vi "Refactor Class Dynamic Dispatch Membersvi.vi"(8 "error in (no error)":errorcluster, 10 "rename data in":T1, 11 "project classes in":refnum<vi>[](array[refnum])) -> (0 "error out":errorcluster, 1 "refactor results":T3[](array[typedef]), 2 "rename metadata out":T1, 3 "project classes out":refnum<vi>[](array[refnum]))   [LabVIEW 2020, in "MeasurementService Editor.lvlib"]
uses:
  MeasurementService Editor.lvlib
  Rename Refactor Data.ctl
  Rename Refactor Mapping Info.ctl
  Refactor Dynamic Dispatch Member Result.ctl
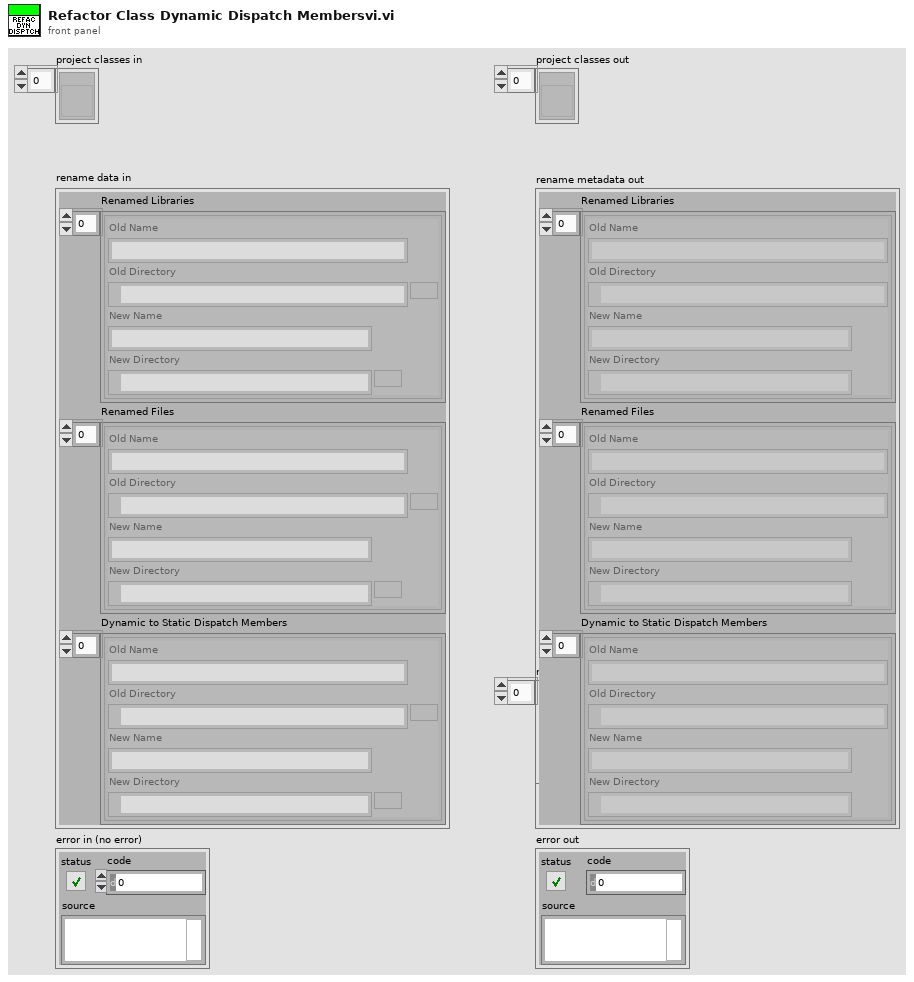
[diagram p1: front panel]
types:
  T1 = typedef "MeasurementService Editor.lvlib/Rename Refactor Data.ctl" = cluster{"Renamed Libraries":T2[], "Renamed Files":T2[], "Dynamic to Static Dispatch Members":T2[]}
  T2 = typedef "MeasurementService Editor.lvlib/Rename Refactor Mapping Info.ctl" = cluster{"Old Name":string, "Old Directory":path, "New Name":string, "New Directory":path}
  T3 = typedef "MeasurementService Editor.lvlib/Refactor Dynamic Dispatch Member Result.ctl" = cluster{"Old Path":path, "New Path":path}
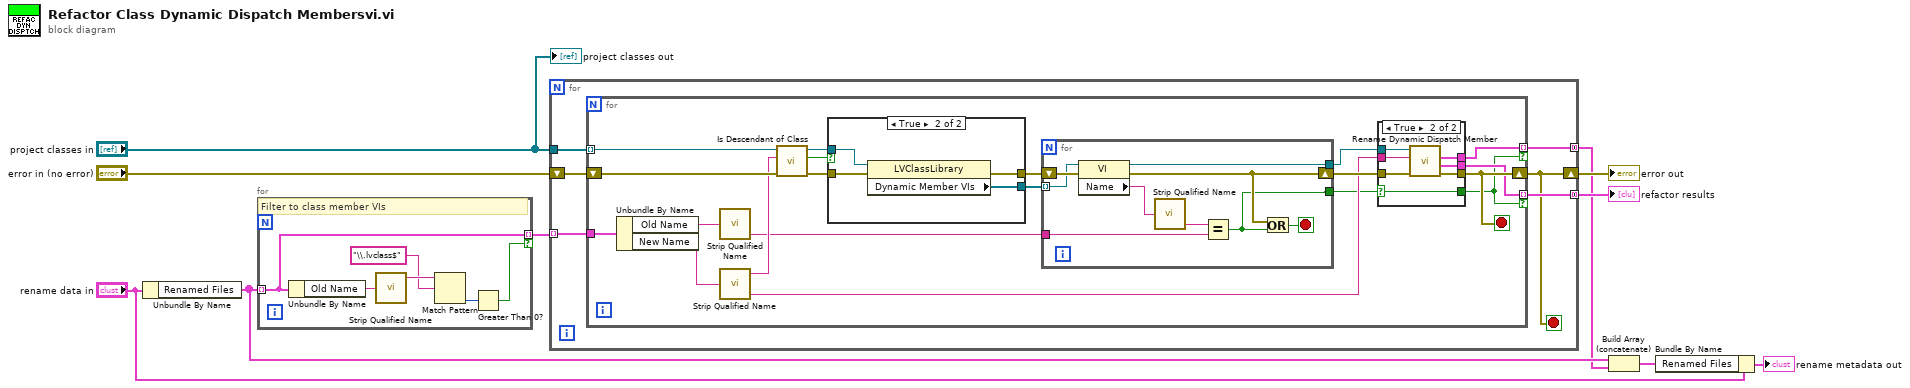
[diagram p0: block diagram]
diagram:
  n1 = Unbundle By Name("rename data in") -> ("Renamed Files"=w5:T2[])
  n2 = for {
    tunnel: w5 -> [w12] mode=indexing
    tunnel: [w12] -> w9 mode=indexing if=w11
    # "Filter to class member VIs"
    n3 = Unbundle By Name(w12) -> ("Old Name"=w16:string)
    n4 = call "Strip Qualified Name.vi"("name"=w16) -> ("stripped name"=w15:string)  [unwired: 5 in, 1 out]
    n5 = Match Pattern(string=w15, regular expression="\\.lvclass$") -> (offset past match=w13:i32)  [unwired: 1 in, 3 out]
    n6 = Greater Than 0?(x=w13) -> (x > 0?=w11:bool)
  }
  n7 = for {
    tunnel: "project classes in" -> [w21]
    tunnel: w9 -> [w22] mode=indexing
    shift-right: [w18] -> w7
    shift-left: "error in (no error)" -> [w20]
    tunnel: [w19] -> w6 mode=concatenating
    tunnel: [w17] -> w4 mode=concatenating
    stop <- w18 stop-if-true
    n8 = for {
      tunnel: w22 -> [w42]
      tunnel: w21 -> [w40] mode=indexing
      shift-right: [w29] -> w18
      shift-left: w20 -> [w39]
      tunnel: [w27] -> w19 mode=indexing if=w23
      tunnel: [w26] -> w17 mode=indexing if=w23
      stop <- w29 stop-if-true
      n9 = Unbundle By Name(w42) -> ("Old Name"=w34:string, "New Name"=w41:string)
      n10 = call "Strip Qualified Name.vi"("name"=w34) -> ("last name"=w28:string)  [unwired: 5 in, 1 out]
      n11 = call "Strip Qualified Name.vi"("name"=w41) -> ("stripped name"=w38:string, "last name"=w25:string)  [unwired: 5 in]
      n12 = call "Is Descendant of Class.vi"("error in (no error)"=w39, "ancestor name"=w38, "class in"=w40) -> ("error out"=w36:errorcluster, "is descendant?"=w35:bool, "class out"=w37:refnum<vi>)  [unwired: 6 in]
      n13 = case shown="True" w35 {
        tunnel: w37 -> [_ w64]
        tunnel: w36 -> [w60 w63]
        tunnel: [w60 w62] -> w33
        tunnel: [_ w61] -> w32
        frame False {
        }
        frame True {
          n14 = property class="LVClassLibrary"(reference=w64, error in=w63) -> (error out=w62:errorcluster, "Dynamic Member VIs"=w61:refnum<vi>[])  [unwired: 1 out]
        }
      }
      n15 = for {
        tunnel: w32 -> [w58] mode=indexing
        shift-right: [w55] -> w31
        shift-left: w33 -> [w59]
        tunnel: w28 -> [w57]
        tunnel: [w54] -> w24
        tunnel: [w53] -> w30
        stop <- w56 stop-if-true
        n16 = property class="VI"(reference=w58, error in=w59) -> (reference out=w53:refnum<vi>, error out=w55:errorcluster, "Name"=w51:string)
        n17 = call "Strip Qualified Name.vi"("name"=w51) -> ("last name"=w52:string)  [unwired: 5 in, 1 out]
        n18 = Equal?(x=w52, y=w57) -> (x = y?=w54:bool)
        n19 = Or(x=w55, y=w54) -> (x .or. y?=w56:bool)
      }
      n20 = case shown="True" w24 {
        selector: w24 -> [_ w44]
        tunnel: w31 -> [w43 w50]
        tunnel: w30 -> [_ w49]
        tunnel: [w43 w48] -> w29
        tunnel: [_ w47] -> w27
        tunnel: [_ w46] -> w26
        tunnel: w25 -> [_ w45]
        tunnel: [_ w44] -> w23
        frame False {
        }
        frame True {
          n21 = call "Rename Dynamic Dispatch Member.vi"("error in (no error)"=w50, "new name"=w45, "vi in"=w49) -> ("error out"=w48:errorcluster, "refactor result"=w47:T3, "additional mapping info"=w46:T2)  [unwired: 6 in]
        }
      }
    }
  }
  "error out" <- w7
  "refactor results" <- w6
  n22 = Build Array (concatenate)(w5, w4) -> (w2:T2[])
  n23 = Bundle By Name(cluster="rename data in", "Renamed Files"=w2) -> (→"rename metadata out":T1)
  "project classes out" <- "project classes in"
